vi "Test Write I32 to Config from Multiple open References.vi"(8 "error in (no error)":errorcluster, 11 "Test Case In":refnum<class "Configuration File Race Condition Test.lvclass">) -> (0 "error out":errorcluster, 3 "Test Case Out":refnum<class "Configuration File Race Condition Test.lvclass">)   [LabVIEW 2020, in "Configuration File Race Condition Test.lvclass"]
uses:
  Configuration File Race Condition Test.lvclass
  Configuration File Race Condition Test.lvclass/Configuration File Race Condition Test.ctl
  01074fa8-ee8a-411d-bc8b-fc92c4f90959.vi
  Mock Configurable Base/Mock Configurable Base.lvclass
panel:
  out "text":string
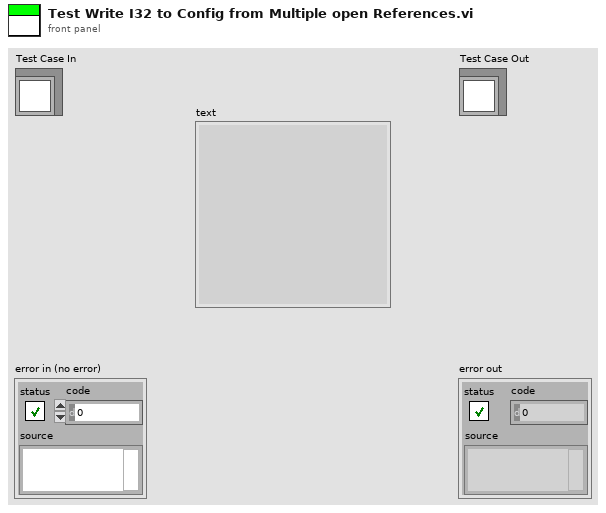
[diagram p1: front panel]
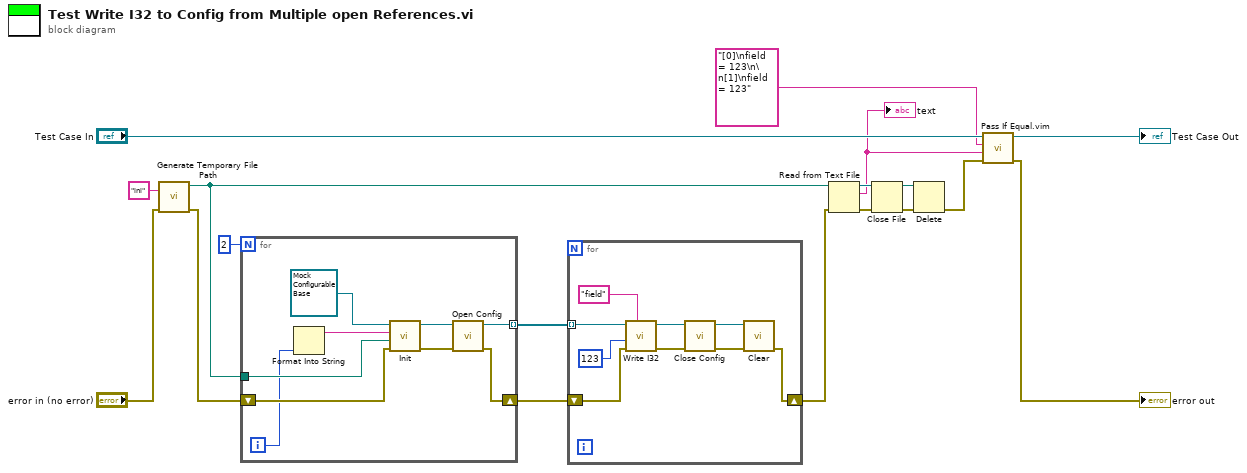
[diagram p0: block diagram]
diagram:
  n1 = call <vilib>:"Generate Temporary File Path.vi"("error in (no error)"="error in (no error)", "Temporary File Extension (tmp)"="ini") -> ("error out"=w14:errorcluster, "Unique Temporary File Path"=w9:path)  [unwired: 8 in]
  n2 = for {
    N: 2 -> [_]
    tunnel: w9 -> [w27]
    shift-right: [w20] -> w11
    shift-left: w14 -> [w25]
    tunnel: [w19] -> w10 mode=indexing
    i -> [w24]
    n3 = Format Into String(w24) -> (resulting string=w23:string)  [unwired: 3 in, 1 out]
    n4 = call-dynamic "Init.vi"("error in (no error)"=w25, "Config File Path"=w27, "Name"=w23, "Base In"=refnum<class "Mock Configurable Base.lvclass"> refnum ("Mock Configurable Base.lvclass")) -> ("error out"=w21:errorcluster, "Base Out"=w22:refnum<class "Mock Configurable Base.lvclass">)  [unwired: 6 in]
    n5 = call-dynamic "Open Config.vi"("error in (no error)"=w21, "Configuration File File In"=w22) -> ("error out"=w20:errorcluster, "Configuration File File Out"=w19:refnum<class "Mock Configurable Base.lvclass">)  [unwired: 8 in]
  }
  n6 = for {
    shift-right: [w30] -> w6
    shift-left: w11 -> [w36]
    tunnel: w10 -> [w35] mode=indexing
    n7 = call-dynamic "Write I32.vi"("key"="field", "error in (no error)"=w36, "Value"=123, "Configuration File In"=w35) -> ("error out"=w33:errorcluster, "Configuration File Out"=w34:refnum<class "Mock Configurable Base.lvclass">)  [unwired: 6 in]
    n8 = call-dynamic "Close Config.vi"("error in (no error)"=w33, "Configuration File File In"=w34) -> ("error out"=w31:errorcluster, "Configuration File File Out"=w32:refnum<class "Mock Configurable Base.lvclass">)  [unwired: 8 in]
    n9 = call-dynamic "Clear.vi"("error in (no error)"=w31, "Base In"=w32) -> ("error out"=w30:errorcluster)  [unwired: 9 in]
  }
  n10 = Read from Text File(file (use dialog)=w9, error in=w6) -> (refnum out=w7:refnum<file>, text=w4:string, error out=w8:errorcluster)  [unwired: 2 in, 1 out]
  "text" <- w4
  n11 = Close File(refnum=w7, error in=w8) -> (path=w1:path, error out=w5:errorcluster)
  n12 = Delete(path (use dialog)=w1, error in=w5) -> (error out=w2:errorcluster)  [unwired: 3 in, 2 out]
  n13 = call "Pass If Equal.vim"("error in (no error)"=w2, "Actual"=w4, "Expected"="[0]\nfield = 123\n\n[1]\nfield = 123" ("text"), "LUnit Test Case In"="Test Case In") -> ("error out"=→"error out":errorcluster, "LUnit Test Case Out"=→"Test Case Out":refnum<class "Configuration File Race Condition Test.lvclass">)  [unwired: 6 in]
